vi "POST (Multipart).vi"(6 "timeout":i32=10000, 7 "output file":path, 8 "error in":errorcluster, 9 "Multipart Post data":T1[](array[typedef]), 10 "url":string, 11 "http-method in":refnum<class "http-client.lvclass">) -> (0 "error out":errorcluster, 2 "response":refnum<class "response.lvclass">, 3 "http-method out":refnum<class "http-client.lvclass">)   [LabVIEW 2020, in "http.lvlib" / "http-client.lvclass"]
uses:
  http-client.lvclass
  response/response.lvclass
  <vilib>/httpClient/MultipartData.ctl
  <vilib>/httpClient/LabVIEWHTTPClient.lvlib
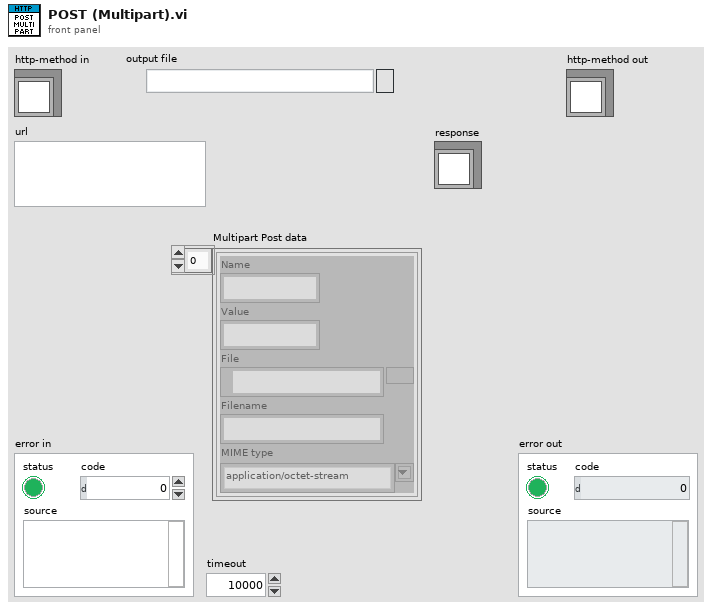
[diagram p1: front panel]
types:
  T1 = typedef "LabVIEWHTTPClient.lvlib/MultipartData.ctl" = cluster{"Name":string, "Value":string, "File":path, "Filename":string, "MIME type":string}
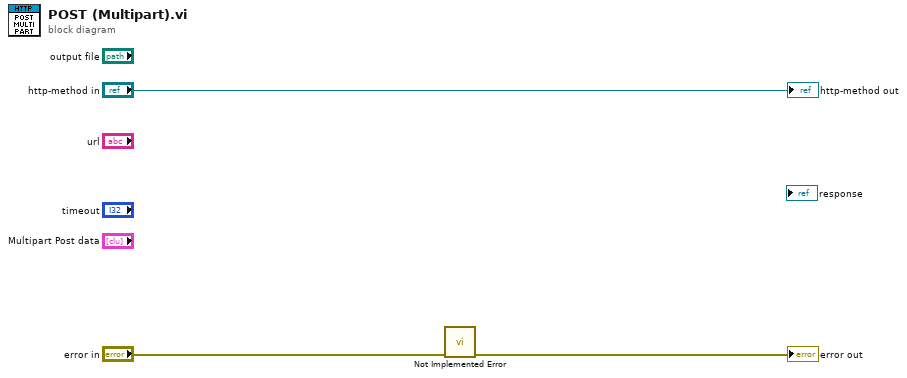
[diagram p0: block diagram]
diagram:
  n1 = call "Not Implemented Error.vi"("error in (no error)"="error in") -> ("error out"=→"error out":errorcluster)  [unwired: 10 in]
  "http-method out" <- "http-method in"
